vi "Write Response.vi"(6 "overwrite on timeout (T)":bool, 8 "error in (no error)":errorcluster, 9 "timeout in ms (0)":i32, 10 "response":T1, 11 "Interface in":refnum<class "Interface.lvclass">) -> (0 "error out":errorcluster, 1 "timed out?":bool, 3 "Interface out":refnum<class "Interface.lvclass">)   [LabVIEW 2017, in "DSF Core.lvlib" / "Interface.lvclass"]
uses:
  Interface.lvclass
  RT FIFO Data 16B.ctl
  RT FIFO Payload 16B.ctl
  Interface.lvclass/Interface.ctl
  Debug/FIFO Flags/FIFO Flags.lvclass/FIFO Flags.ctl
  Debug/FIFO Flags/Get Infinite Timeouts.vi
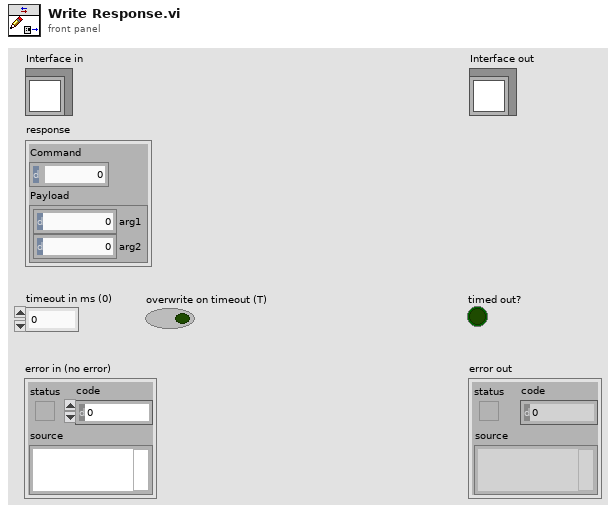
[diagram p1: front panel]
types:
  T1 = typedef "DSF Core.lvlib/Interface.lvclass/RT FIFO Data 16B.ctl" = cluster{"Command":u8, "Payload":T2}
  T2 = typedef "DSF Core.lvlib/Interface.lvclass/RT FIFO Payload 16B.ctl" = cluster{"arg1":u64, "arg2":u64}
  T3 = typedef "DSF Core.lvlib/Interface.lvclass/RT FIFO Ref 16B.ctl" = refnum<k33>
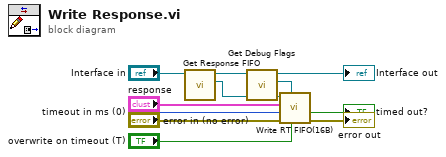
[diagram p0: block diagram]
diagram:
  n1 = call "Get Response FIFO.vi"("Interface in"="Interface in") -> ("Response FIFO"=w11:T3, "Interface out"=w7:refnum<class "Interface.lvclass">)  [unwired: 9 in]
  n2 = call "Get Debug Flags.vi"("Interface in"=w7) -> ("FIFO Debug Flags"=w6:refnum<class "FIFO Flags.lvclass">, "Interface out"=→"Interface out":refnum<class "Interface.lvclass">)  [unwired: 9 in]
  n3 = call "Write RT FIFO(16B).vi"("overwrite on timeout (T)"="overwrite on timeout (T)", "FIFO Debug Flags"=w6, "error in (no error)"="error in (no error)", "timeout in ms (0)"="timeout in ms (0)", "element"="response", "RT FIFO in"=w11) -> ("error out"=→"error out":errorcluster, "timed out?"=→"timed out?":bool)  [unwired: 3 in, 1 out]
